vi "Calculate dt.vi"(8 "error in":errorcluster, 9 "Voltage in":waveform(dbl)[](array[waveform]), 10 "t_start in":dbl, 11 "dt in":dbl) -> (0 "error out":errorcluster, 3 "t_start out":dbl)   [LabVIEW 2021]
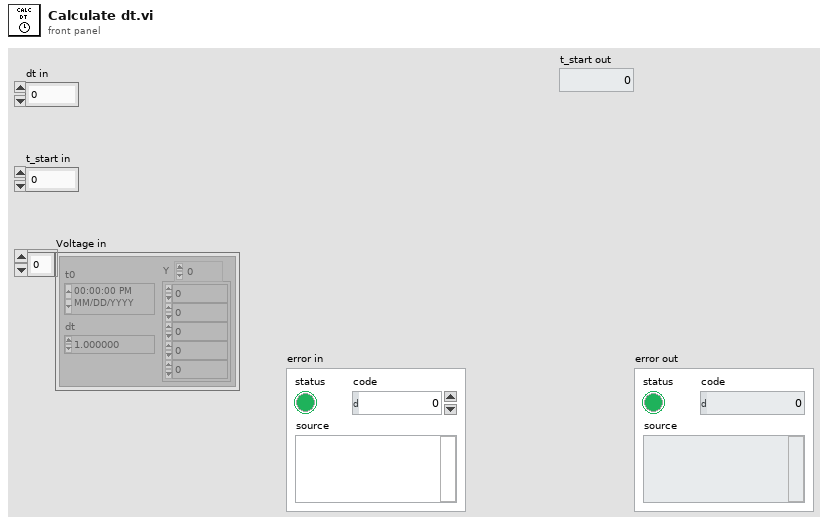
[diagram p1: front panel]
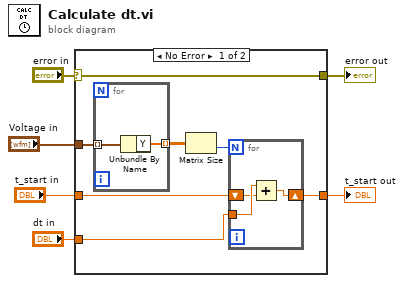
[diagram p0: block diagram]
diagram:
  n1 = case shown="No Error" "error in" {
    selector: "error in" -> [w13 w20]
    tunnel: [w13 w20] -> w5
    tunnel: "Voltage in" -> [w12 _]
    tunnel: "t_start in" -> [w9 w19]
    tunnel: "dt in" -> [w8 _]
    tunnel: [w7 w19] -> w1
    frame No Error {
      n2 = for {
        tunnel: w12 -> [w17] mode=indexing
        tunnel: [w18] -> w11 mode=indexing
        n3 = Unbundle By Name(w17) -> ("Y"=w18:dbl[])
      }
      n4 = Matrix Size(0:w11) -> (2:w10:i32)  [unwired: 1 out]
      n5 = for {
        N: w10 -> [_]
        tunnel: w8 -> [w15]
        shift-right: [w16] -> w7
        shift-left: w9 -> [w14]
        n6 = Add(x=w15, y=w14) -> (x+y=w16:dbl)
      }
    }
    frame Error {
    }
  }
  "error out" <- w5
  "t_start out" <- w1
